vi "test_parseCcdData.vi"(8 "error in (no error)":errorcluster) -> (0 "error out":errorcluster)   [LabVIEW 2023, in "horiba.test.lvlib"]
uses:
  horiba.test.lvlib
  Classes/CCD/ccdAcquisitionData.ctl
  Classes/CCD/imageAcqData.ctl
  Classes/CCD/roiMetaData.ctl
  <vilib>/addons/_JKI Toolkits/Caraya/classes/Assert/Assert Equal Value and Type_Variant.vi
  <vilib>/addons/_JKI Toolkits/Caraya/classes/Assert/Assert Not Error.vi
  <vilib>/addons/_JKI Toolkits/Caraya/classes/Test/Test.lvclass
  <vilib>/addons/_JKI Toolkits/Caraya/classes/Assert/Assert.lvclass
  Classes/CCD/CCD.lvclass
panel:
  # "Connector Pane"
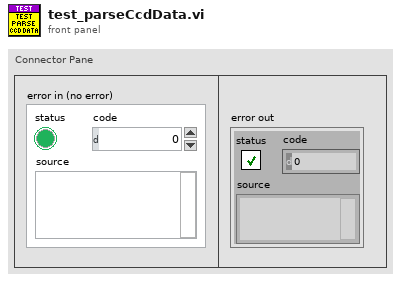
[diagram p1: front panel]
types:
  T1 = typedef "horiba.lvlib/CCD.lvclass/ccdAcquisitionData.ctl" = cluster{"acqIndex":i32, "ROIs":T2[], "timestamp":string}
  T2 = typedef "horiba.lvlib/CCD.lvclass/imageAcqData.ctl" = cluster{"roiMetaData":T3, "xAxis":dbl[], "yData":dbl[][]}
  T3 = typedef "horiba.lvlib/CCD.lvclass/roiMetaData.ctl" = cluster{"roiIndex":i32, "xBinning":i32, "xOrigin":i32, "xSize":i32, "yBinning":i32, "yOrigin":i32, "ySize":i32}
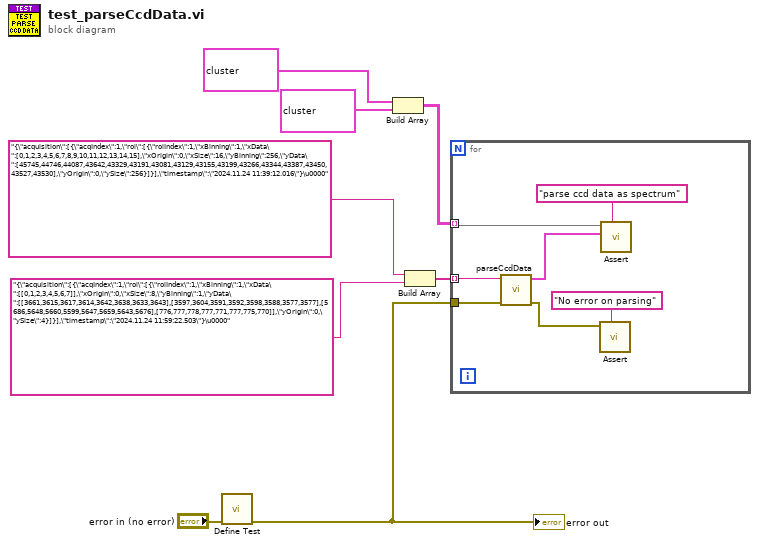
[diagram p0: block diagram]
diagram:
  n1 = call <vilib>:"Define Test.vi"("error in (no error)"="error in (no error)") -> ("error out"=w7:errorcluster)  [unwired: 9 in, 1 out]
  "error out" <- w7
  n2 = Build Array(T1[] [{"acqIndex"=1, "ROIs"=[{"roiMetaData"={"roiIndex"=1, "xBinning"=1, "xOrigin"=0, "xSize"=16, "yBinning"=256, "yOrigin"=0, "ySize"=256}, "xAxis"=[0.0, 1.0, 2.0, 3.0, 4.0, 5.0, 6.0, 7.0, 8.0, 9.0, 10.0, 11.0, 12.0, 13.0, 14.0, 15.0], "yData"=[[45745.0, 44746.0, 44087.0, 43642.0, 43329.0, 43191.0, 43081.0, 43129.0, 43155.0, 43199.0, 43266.0, 43344.0, 43387.0, 43450.0, 43527.0, 43530.0]]}], "timestamp"="\"2024.11.24 11:39:12.016\""}] ("ccdData"), T1[] [{"acqIndex"=1, "ROIs"=[{"roiMetaData"={"roiIndex"=1, "xBinning"=1, "xOrigin"=0, "xSize"=8, "yBinning"=1, "yOrigin"=0, "ySize"=4}, "xAxis"=[0.0, 1.0, 2.0, 3.0, 4.0, 5.0, 6.0, 7.0], "yData"=[[3661.0, 3597.0, 5686.0, 776.0], [3615.0, 3604.0, 5648.0, 777.0], [3617.0, 3591.0, 5660.0, 778.0], [3614.0, 3592.0, 5599.0, 777.0], [3642.0, 3598.0, 5647.0, 771.0], [3638.0, 3588.0, 5659.0, 777.0], [3633.0, 3577.0, 5643.0, 775.0], [3643.0, 3577.0, 5676.0, 770.0]]}], "timestamp"="\"2024.11.24 11:59:22.503\""}] ("ccdData")) -> (w3:T1[][])
  n3 = Build Array("{\"acquisition\":[{\"acqIndex\":1,\"roi\":[{\"roiIndex\":1,\"xBinning\":1,\"xData\":[0,1,2,3,4,5,6,7,8,9,10,11,12,13,14,15],\"xOrigin\":0,\"xSize\":16,\"yBinning\":256,\"yData\":[45745,44746,44087,43642,43329,43191,43081,43129,43155,43199,43266,43344,43387,43450,43527,43530],\"yOrigin\":0,\"ySize\":256}]}],\"timestamp\":\"2024.11.24 11:39:12.016\"}\u0000" ("results-JSON string"), "{\"acquisition\":[{\"acqIndex\":1,\"roi\":[{\"roiIndex\":1,\"xBinning\":1,\"xData\":[[0,1,2,3,4,5,6,7]],\"xOrigin\":0,\"xSize\":8,\"yBinning\":1,\"yData\":[[3661,3615,3617,3614,3642,3638,3633,3643],[3597,3604,3591,3592,3598,3588,3577,3577],[5686,5648,5660,5599,5647,5659,5643,5676],[776,777,778,777,771,777,775,770]],\"yOrigin\":0,\"ySize\":4}]}],\"timestamp\":\"2024.11.24 11:59:22.503\"}\u0000" ("results-JSON string")) -> (w5:string[])
  n4 = for {
    tunnel: w5 -> [w14] mode=indexing
    tunnel: w7 -> [w15]
    tunnel: w3 -> [w9] mode=indexing
    n5 = call "parseCcdData.vi"("error in (no error)"=w15, "results-JSON string"=w14) -> ("error out"=w13:errorcluster, "ccdData"=w10:T1[])  [unwired: 8 in]
    n6 = call-poly <vilib>:"Assert.vi"("Label"="No error on parsing", "Not Error?"=w13) -> ()  [unwired: 8 in, 2 out]
    n7 = call-poly <vilib>:"Assert.vi"("Label"="parse ccd data as spectrum" ("Label (VI Title)"), "Y"=w10, "X"=w9) -> ()  [unwired: 7 in, 2 out]
  }
